vi "ConfigureChannel.vi"(4 "Initial value":bool, 5 "Direction":T2, 6 "Pull up/down":T1, 7 "Channel":i32, 8 "error in":errorcluster) -> (0 "error out":errorcluster)   [LabVIEW 2014, in "GPIO.lvlib"]
doc: "Confgure a single channel as either an input or output. For inputs you can also specify the software pull up/down. For outputs you can provide an initial value.\n\nThis VO must be called before reading from or writing to a channel."
uses:
  GPIO.lvlib
  controls/IO_Direction.ctl
  controls/PullUpDown.ctl
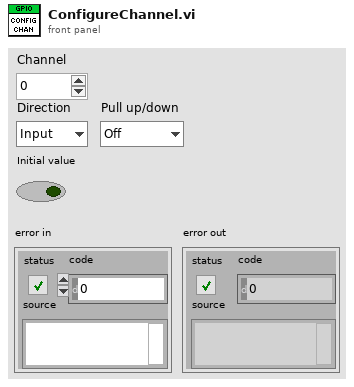
[diagram p1: front panel]
types:
  T1 = typedef "GPIO.lvlib/PullUpDown.ctl" = enum16{"Off", "Pull up", "Pull down"}
  T2 = typedef "GPIO.lvlib/IO_Direction.ctl" = enum16{"Input", "Output"}
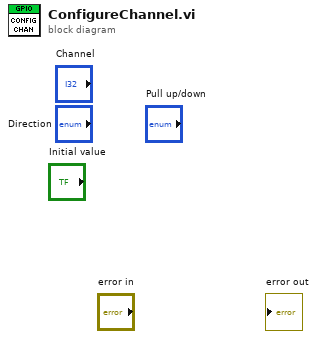
[diagram p0: block diagram]
diagram:
